vi "PH_Stepmotor_BaseClass.PC set Position in Units.vi"(0 "i ref in":refnum<vi>, 1 "axis":i32=-1, 2 "Position to set [Units]":dbl, 3 "Set?":bool, 5 "error in (no error)":errorcluster) -> (14 "i ref out":refnum<vi>, 16 "ok?":bool, 19 "error out":errorcluster)   [LabVIEW 2014, in "PH_Stepmotor_BaseClass.lvlib"]
doc: "This VI stores the position in own attributes and sets a flag."
uses:
  PH_Stepmotor_BaseClass.lvlib
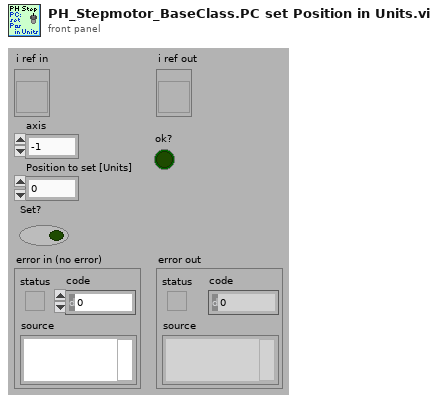
[diagram p1: front panel]
types:
  T1 = typedef "PH_Stepmotor_BaseClass.lvlib/PH_Stepmotor_BaseClass.Axis Attributes.ctl" = cluster{"Settings":T2, "Endswitch?":bool, "DIM Service IDs":T4, "Activity":T5, "Configured?":bool, "Position":cluster{"Current":i32, "Target":i32}, "Position to set":cluster{"New?":bool, "Wanted":i32}, "Stop?":bool, "Reset?":bool, "Move?":bool, "Nothing connected?":bool}
  T2 = typedef "PH_Stepmotor_BaseClass.lvlib/PH_Stepmotor_BaseClass.Axis Settings.ctl" = cluster{"Sign change":bool, "Width":dbl, "Calibration":dbl, "Unit":string, "Motor Type":T3, "Unit Width":string, "Unit CF":string}
  T3 = typedef "PH_Stepmotor_BaseClass.lvlib/PH_Stepmotor_BaseClass.Motor Type.ctl" = enum16{"Unspecific", "OWIS 49.120.2633", "OWIS 49.060.1033", "OWIS 43.040.2558", "Diamond Motion 2200 series", "OWIS 49.120.266B.MV6", "Calorimeter", "Linear Stage 1", "MICOS VT-80", "MICOS VT-80 S", "Standa Rotstage nt0.95A", "PUF RA 320.200", "PUF RA 800.200", "PUF RA 800.400", "PUF RA 400.50", "1324.nn.800.50", "1324.n9c.800.50", "1324.nn.320.200", "1324.nn.400.200", "1324.nn.800.200", "1324.nn.400.50", "1324.8c9c.800.50", "1324.8c9c.400.200"}
  T4 = typedef "PH_Stepmotor_BaseClass.lvlib/PH_Stepmotor_BaseClass.Axis DIM Service IDs.ctl" = cluster{"Settings":i32, "Information":i32}
  T5 = typedef "PH_Stepmotor_BaseClass.lvlib/PH_Stepmotor_BaseClass.Axis Activity.ctl" = enum16{"No Information", "stopped", "running", "Failure", "Alarm", "stopped at backward ES", "stopped at foreward ES"}
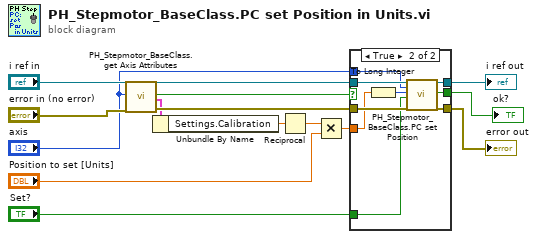
[diagram p0: block diagram]
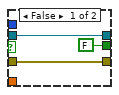
[diagram p2: hidden frame]
diagram:
  n1 = call "PH_Stepmotor_BaseClass.get Axis Attributes.vi"("VI in"="i ref in", "Axis"="axis", "error in (no error)"="error in (no error)") -> ("VI out"=w11:refnum<vi>, "Axis found?"=w3:bool, "Axis Attributes"=w10:T1, "error out"=w12:errorcluster)  [unwired: 13 in]
  n2 = Unbundle By Name(w10) -> ("Settings.Calibration"=w7:dbl)
  n3 = Reciprocal(x=w7) -> (1/x=w6:dbl)
  n4 = Multiply(x=w6, y="Position to set [Units]") -> (x*y=w4:dbl)
  n5 = case shown="True" w3 {
    tunnel: [w18 w27] -> w14
    tunnel: [w17 w26] -> w13
    tunnel: w12 -> [w17 w25]
    tunnel: w11 -> [w18 w24]
    tunnel: [FALSE ("ok?") w23] -> w9
    tunnel: "Set?" -> [_ w22]
    tunnel: w4 -> [_ w21]
    tunnel: "axis" -> [_ w19]
    frame False {
    }
    frame True {
      n6 = To Long Integer(number=w21) -> (32bit integer=w20:i32)
      n7 = call "PH_Stepmotor_BaseClass.PC set Position.vi"("i ref in"=w24, "axis"=w19, "Position to set"=w20, "Set?"=w22, "error in (no error)"=w25) -> ("i ref out"=w27:refnum<vi>, "ok?"=w23:bool, "error out"=w26:errorcluster)  [unwired: 12 in]
    }
  }
  "error out" <- w13
  "i ref out" <- w14
  "ok?" <- w9
